vi "TOOLweb SET LABFILE Enabled.vi"(4 "error in (no error)":errorcluster, 5 "IP-Adresse (localhost)":string="127.0.0.1", 7 "Enabled":bool) -> (1 "Feedback":i32)   [LabVIEW 2020]
doc: "Aktiviert das Speichern von Spektren in \"labfiles\" mit einem SET-Request (EVID 80).\nTRUE = labEnabled, FALSE = labDisabled.\nDer Integer-Ausgang \"Feedback\" gibt Auskunft über die erfolgreiche Ausführung des Set-Requests, wobei nur der Wert 0 (=success) für alle EVIDs gleich ist. Fehlermeldungen in Form einer Feedback-Zahl ungleich Null variieren und müssen mit dem Handbuch des Gas-Analysators interpretiert werden.\n\nFalls der TOOLWeb-Server nicht auf demselben Rechner arbeitet, kann mit \"IP-Adresse\" eine beliebiger Host adressiert werden. Ein unverbundener Eingang spricht den lokalen Host an."
uses:
  Stoerungen/Stoerungen Messgeraet/Aktionen Kommunikation Stoerung.ctl
  Log Konfig/Aktion LabBaseIndex.ctl
  FGV FT-IR Aktionen.ctl
  TOOLweb Interface.lvlib
  Stoerungen/Stoerungen.lvlib
  FT-IR.lvlib
  Log Konfig/LogKonfig.lvlib
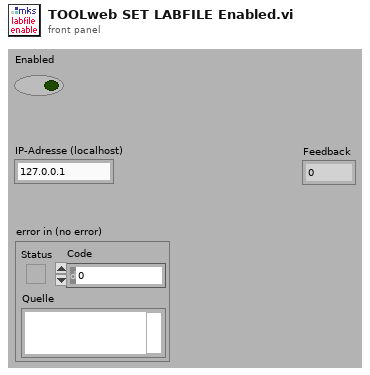
[diagram p1: front panel]
types:
  T1 = typedef "Stoerungen.lvlib/Aktionen Kommunikation Stoerung.ctl" = enum16{"lesen", "init", "FT-IR Komm", "FT-IR Betriebsart", "FT-IR Hintergrund", "cRIO Komm", "PNS Komm", "Dichtheitstest", "Life Bit", "FTIR Komm AK", "PMA Komm", "FID Komm", "PMA Cal", "FID Ch4 Cal", "FID THC Cal", "Cal Timeout", "VFS 1 Komm", "VFS 2 Komm", "VFS 3 Komm", "VFS 4 Komm", "TRE 08 Komm", "CG-Test vorzeitig", "CG-Test Span 1", "CG-Test Span 2", "CG-Test Span 3", "CG-Test Messgas", "CG-Test löschen", "Test", "Amium AK", "AK Recept konfig", "AK Name konfig", "AK EKFG konfig"}
  T2 = typedef "LogKonfig.lvlib/Aktion LabBaseIndex.ctl" = enum16{"lesen", "schreiben"}
  T3 = typedef "FT-IR.lvlib/FGV FT-IR Aktionen.ctl" = enum16{"lesen", "NOG setzen", "NOS setzen", "Initialisieren", "speichern", "ALLES setzen", "FT-IR Spektrum loggen", "Komm Stoppen", "Spektrum LogKonfig"}
  T4 = cluster{"(80) labEnabled":bool, "(81) labPath":path, "(82) labBaseName":string, "(83) labIndex":string, "Spektrum loggen aktiv?":bool}
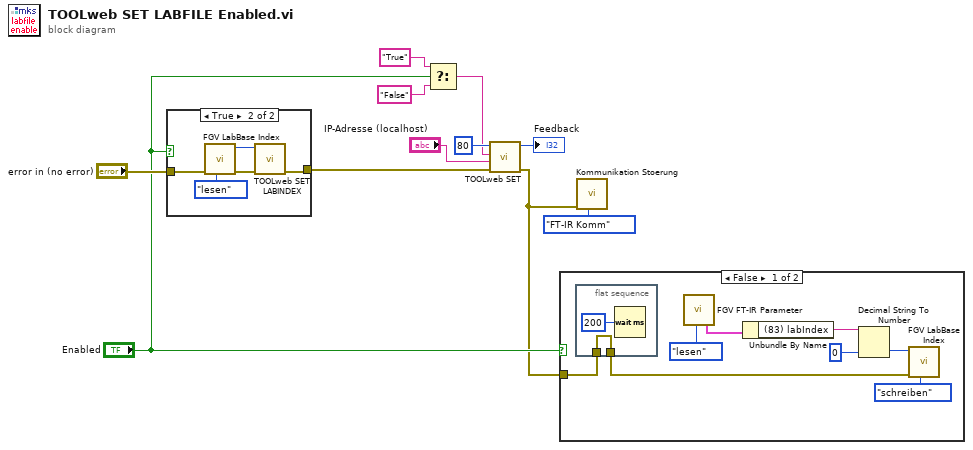
[diagram p0: block diagram]
diagram:
  n1 = case shown="True" "Enabled" {
    tunnel: "error in (no error)" -> [w12 w15]
    tunnel: [w12 w13] -> w3
    frame False {
    }
    frame True {
      n2 = call "FGV LabBase Index.vi"("Aktion"=Aktion_LabBaseIndex."lesen", "error in (no error)"=w15) -> ("error out"=w14:errorcluster, "Index Nr. Start:"=w17:u32)  [unwired: 8 in]
      n3 = call "TOOLweb SET LABINDEX.vi"("error in (no error)"=w14, "SPEC#:"=w17) -> ("error out"=w13:errorcluster)  [unwired: 3 in, 2 out]
    }
  }
  n4 = Select(t="True", s="Enabled", f="False") -> (s? t:f=w7:string)
  n5 = call "TOOLweb SET.vi"("error in (no error)"=w3, "IP-Adresse (localhost)"="IP-Adresse (localhost)", "Wert-String"=w7, "EVID-Nummer"=80) -> ("error out"=w1:errorcluster, "Feedback"=→"Feedback":i32)  [unwired: 2 out]
  n6 = case shown="False" "Enabled" {
    tunnel: w1 -> [w19 _]
    frame False {
      n7 = flat-sequence {
        tunnel: w19 -> [w26]
        tunnel: [w26] -> w18
        frame #0 {
          n8 = Wait (ms)(milliseconds to wait=u32 200 ("Zu wartende ms")) -> ()  [unwired: 1 out]
        }
      }
      n9 = call "FGV FT-IR Parameter.vi"("Aktion"=FGV_FT-IR_Aktionen."lesen") -> ("Ausgangs-Cluster"=w24:T4)  [unwired: 11 in, 7 out]
      n10 = Unbundle By Name(w24) -> ("(83) labIndex"=w22:string)
      n11 = Decimal String To Number(string=w22, default (0L)=u32 0 ("SPEC#:")) -> (number=w21:u32)  [unwired: 1 in, 1 out]
      n12 = call "FGV LabBase Index.vi"("Aktion"=Aktion_LabBaseIndex."schreiben", "error in (no error)"=w18, "Index Nr. Start:"=w21) -> ()  [unwired: 7 in, 2 out]
    }
    frame True {
    }
  }
  n13 = call "Kommunikation Stoerung.vi"("Aktionen"=Aktionen_Kommunikation_Stoerung."FT-IR Komm", "error in"=w1) -> ()  [unwired: 9 in, 1 out]
